vi "IsEvenSGL.vi"(4 "x":sgl) -> (1 "Even?":bool)   [LabVIEW 2017, in "GPComparison.lvlib"]
doc: "<B>Even?</B> will be True if <B>x</B> is an even integer.\n\nThis VI is inlined.\n\nSteen Schmidt\nGPower\n6/3 2013"
uses:
  GPComparison.lvlib
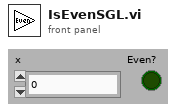
[diagram p1: front panel]
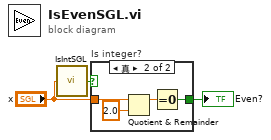
[diagram p0: block diagram]
diagram:
  n1 = call "IsIntSGL.vi"("x"="x") -> ("Integer?"=w2:bool)  [unwired: 4 in]
  n2 = case "Is integer?" shown="真" w2 {
    tunnel: [_ w4] -> w3
    tunnel: "x" -> [_ w7]
    frame False {
    }
    frame True {
      n3 = Quotient & Remainder(x=w7, y=sgl 2.0) -> (x-y*floor(x/y)=w5:sgl)  [unwired: 1 out]
      n4 = Equal To 0?(x=w5) -> (x = 0?=w4:bool)
    }
  }
  "Even?" <- w3
